vi "EDGE TEST.vi"   [LabVIEW 2016, in "Test2.lvrbt"]
uses:
  Test2.lvrbt
  <vilib>/NXT/Block Support/NXT_InputPort.ctl
  <vilib>/NXT/Hardware/Plugins/Tetrix DC Motor/TetrixDCMotorAddress.ctl
  <vilib>/NXT/Dual Mode Library/Sensors/EV3_Ultrasonic_CM.vi
  <vilib>/NXT/NXTIO Xnodes/NXTIONodeSubVIs/TETRIX IO Move DC Motors.vi
  <vilib>/NXT/NXTIO Xnodes/NXTIONodeSubVIs/TETRIX IO Stop DC Motors.vi
  <vilib>/NXT/Dual Mode Library/Waits/Wait_Num.vi
  <vilib>/NXT/NXTIO Xnodes/AddressXNode/NXTIOAddress.xnode
  <vilib>/NXT/Subs/LVHSConnector.ctl
  <vilib>/NXT/NXTIO Xnodes/NXTIOXNode/NXTIO.xnode
  <vilib>/NXT/LegoClasses/BrickReference/BrickReference.lvclass
types:
  T1 = typedef "TetrixDCMotorAddress.ctl" = i32
  T2 = cluster{"TetrixDCMotor":T1, "TetrixDCMotor 2":T1}
  T3 = typedef "NXT_InputPort.ctl" = u32
  T4 = typedef "LVHSConnector.ctl" = refnum<class "BrickReference.lvclass">
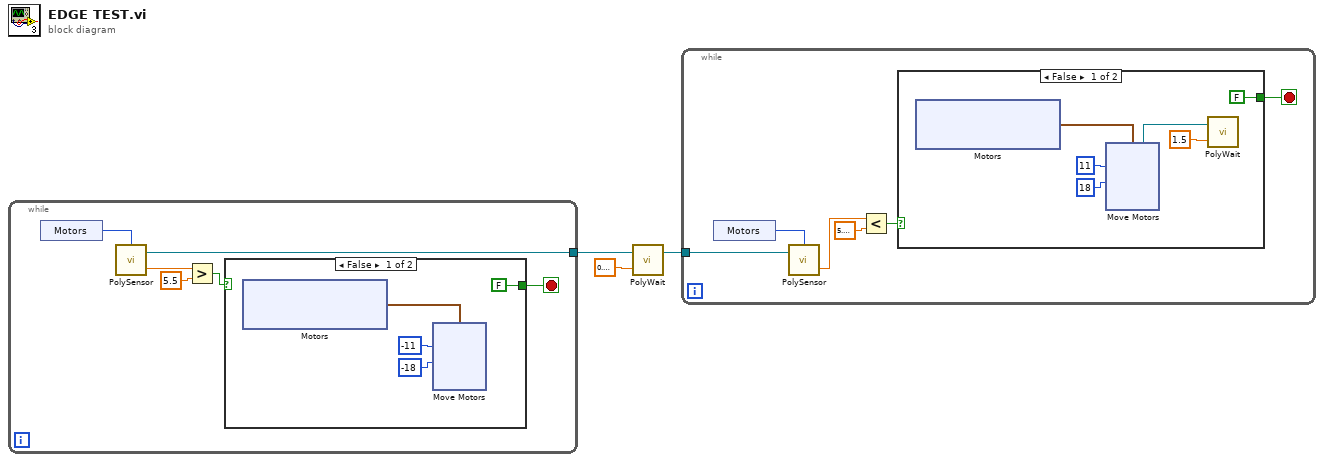
[diagram p0: block diagram]
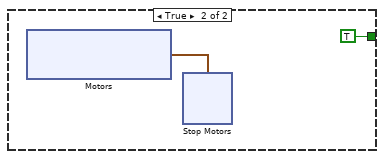
[diagram p2: hidden frame]
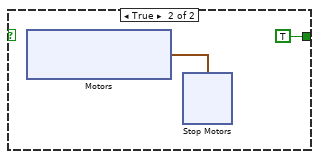
[diagram p3: hidden frame]
diagram:
  n1 = while {
    tunnel: [w4] -> w1
    stop <- w5 stop-if-true
    n2 = xnode "Motors"() -> ("Sensor"=w9:T3)
    n3 = call-poly <vilib>:"PolySensor.vi"("Port (Port 1)"=w9) -> ("Centimeters"=w8:sgl, "NXT/EV3"=w4:T4)  [unwired: 2 in]
    n4 = Greater?(x=w8, y=sgl 5.5) -> (0:w6:bool)
    n5 = case shown="False" w6 {
      tunnel: [FALSE TRUE] -> w5
      frame False {
        n6 = xnode "Motors"() -> ("Motor"=w13:cluster{"TetrixDCMotor":T1, "TetrixDCMotor":T1})
        n7 = xnode "Move Motors"("Power/Speed 2"=i8 -18, "Power/Speed 1"=i8 -11, "Motors"=w13) -> ()  [unwired: 1 in, 1 out]
      }
      frame True {
        n8 = xnode "Motors"() -> ("Motor"=w24:cluster{"TetrixDCMotor":T1, "TetrixDCMotor":T1})
        n9 = xnode "Stop Motors"("Motors"=w24) -> ()  [unwired: 1 in, 1 out]
      }
    }
  }
  n10 = call-poly <vilib>:"PolyWait.vi"("Time (1 sec)"=sgl 0.8, "NXT/EV3"=w1) -> ("NXT/EV3"=w2:T4)  [unwired: 2 in]
  n11 = while {
    tunnel: w2 -> [w37]
    stop <- w34 stop-if-true
    n12 = xnode "Motors"() -> ("Sensor"=w32:T3)
    n13 = call-poly <vilib>:"PolySensor.vi"("NXT/EV3"=w37, "Port (Port 1)"=w32) -> ("Centimeters"=w36:sgl)  [unwired: 1 in, 1 out]
    n14 = Less?(x=w36, y=sgl 5.3) -> (x < y?=w33:bool)
    n15 = case shown="False" w33 {
      tunnel: [FALSE TRUE] -> w34
      frame False {
        n16 = xnode "Motors"() -> ("Motor"=w44:cluster{"TetrixDCMotor":T1, "TetrixDCMotor":T1})
        n17 = xnode "Move Motors"("Power/Speed 2"=i8 18, "Power/Speed 1"=i8 11, "Motors"=w44) -> ("NXT/EV3"=w41:T4)  [unwired: 1 in]
        n18 = call-poly <vilib>:"PolyWait.vi"("Time (1 sec)"=sgl 1.5, "NXT/EV3"=w41) -> ()  [unwired: 2 in, 1 out]
      }
      frame True {
        n19 = xnode "Motors"() -> ("Motor"=w55:cluster{"TetrixDCMotor":T1, "TetrixDCMotor":T1})
        n20 = xnode "Stop Motors"("Motors"=w55) -> ()  [unwired: 1 in, 1 out]
      }
    }
  }
